vi "plugins_find_directory.vi"() -> (2 "file or folder exists?":bool, 3 "dup path":path)   [LabVIEW 2019]
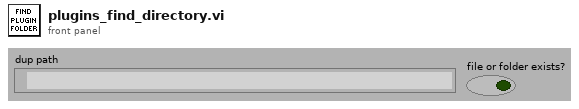
[diagram p1: front panel]
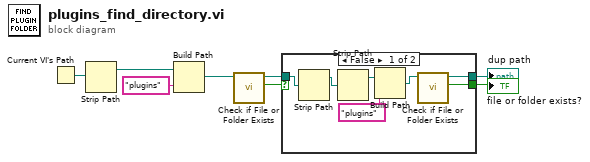
[diagram p0: block diagram]
diagram:
  n1 = Current VI's Path() -> (path=w7:path)
  n2 = Strip Path(path=w7) -> (stripped path=w8:path)  [unwired: 1 out]
  n3 = Build Path(base path=w8, name or relative path="plugins") -> (appended path=w5:path)
  n4 = call <vilib>:"Check if File or Folder Exists.vi"("path"=w5) -> ("file or folder exists?"=w4:bool, "dup path"=w3:path)  [unwired: 8 in, 1 out]
  n5 = case shown="False" w4 {
    selector: w4 -> [_ w16]
    tunnel: w3 -> [w10 w17]
    tunnel: [w12 w17] -> w1
    tunnel: [w11 w16] -> w2
    frame False {
      n6 = Strip Path(path=w10) -> (stripped path=w9:path)  [unwired: 1 out]
      n7 = Strip Path(path=w9) -> (stripped path=w14:path)  [unwired: 1 out]
      n8 = Build Path(base path=w14, name or relative path="plugins") -> (appended path=w13:path)
      n9 = call <vilib>:"Check if File or Folder Exists.vi"("path"=w13) -> ("file or folder exists?"=w11:bool, "dup path"=w12:path)  [unwired: 8 in, 1 out]
    }
    frame True {
    }
  }
  "file or folder exists?" <- w2
  "dup path" <- w1
